vi "dw LP filter.vi"(7 "reset":bool=TRUE, 8 "input valid":bool=TRUE, 11 "x":fxp<+/-,32,14>) -> (0 "output valid":bool, 3 "y":fxp<+/-,32,14>)   [LabVIEW 2018]
uses:
  <vilib>/rvi/Emulation/niFpgaEmulationIsFPGAContextNoSignature.vi
  <vilib>/rvi/DataTransferAndStorage/Container/Common/niFpgaContainerGetUniqueNameForEmu.vi
  <vilib>/rvi/Memory/Memory_Emulation/niFpgaMemoryEmulationCacheClearOnFirstRun.vi
  <vilib>/rvi/Memory/Memory_Emulation/nirvimemoryEmulationManagerCache_MakeExclusive.vi
  <vilib>/rvi/Memory/Memory_Emulation/niFpgaMemoryEmulationValidateCache.vi
  <vilib>/rvi/Memory/Memory_Emulation/nirvimemoryEmulationManagerCache_InsertValue.vi
  <vilib>/Utility/error.llb/Clear Errors.vi
  <vilib>/rvi/Memory/Memory_Emulation/nirvimemoryEmulationManagerCache_ReleaseExclusive.vi
  <vilib>/rvi/Memory/Memory_Emulation/nirvimemoryEmulationManagerCache_GetValue.vi
  <vilib>/rvi/Memory/Memory_Emulation/nirvimemoryEmulationManagerCache_SetValue.vi
  <vilib>/rvi/Emulation/niFpgaProcessEmulError.vi
  <vilib>/rvi/Emulation/niFpgaSctlEmulationGetInTimedLoop.vi
  <vilib>/rvi/DataTransferAndStorage/Container/XNode/niFpgaContainer.xnode
  <vilib>/rvi/DataTransferAndStorage/Register/Emulation/niFpgaRegisterEmulation.vi
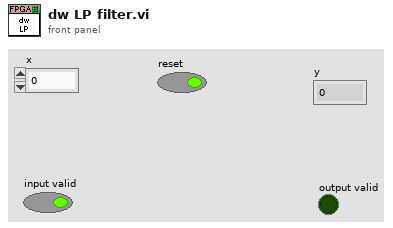
[diagram p1: front panel]
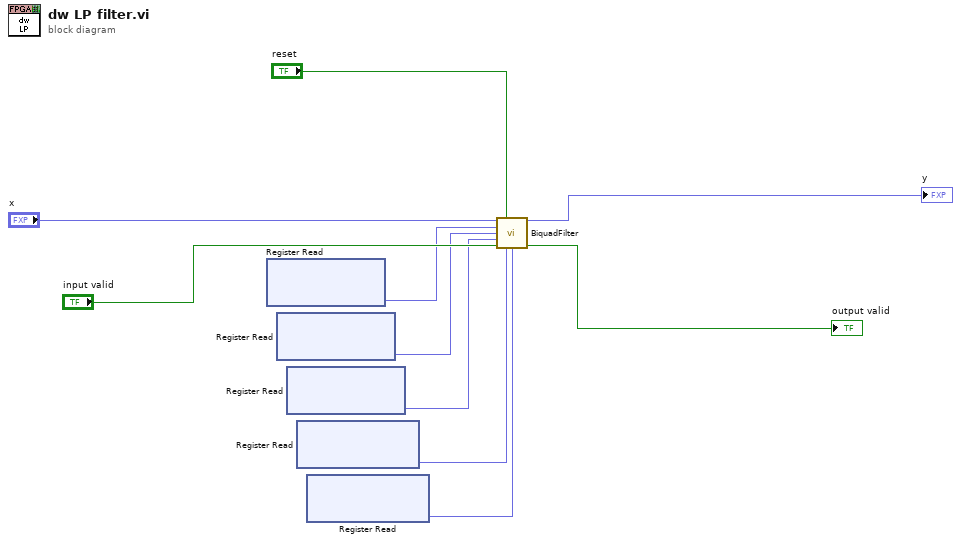
[diagram p0: block diagram]
diagram:
  n1 = xnode "Register Read"() -> ("Data"=w5:fxp<+/-,32,2>)  [unwired: 1 in, 1 out]
  n2 = xnode "Register Read"() -> ("Data"=w4:fxp<+/-,32,2>)  [unwired: 1 in, 1 out]
  n3 = xnode "Register Read"() -> ("Data"=w3:fxp<+/-,32,2>)  [unwired: 1 in, 1 out]
  n4 = xnode "Register Read"() -> ("Data"=w2:fxp<+/-,32,2>)  [unwired: 1 in, 1 out]
  n5 = xnode "Register Read"() -> ("Data"=w1:fxp<+/-,32,2>)  [unwired: 1 in, 1 out]
  n6 = call "BiquadFilter.vi"("x"="x", "reset"="reset", "b0"=w5, "b1"=w4, "b2"=w3, "input valid"="input valid", "-a1"=w2, "-a2"=w1) -> ("y"=→"y":fxp<+/-,32,14>, "output valid"=→"output valid":bool)  [unwired: 6 in]
